vi "Is Concrete Class.vi"(0 "SG 26GHz Path Group in":refnum<class "SG 26GHz Path Group.lvclass">, 11 "error in":errorcluster) -> (4 "SG 26GHz Path Group out":refnum<class "SG 26GHz Path Group.lvclass">, 6 "Is Concrete Class?":bool, 15 "error out":errorcluster)   [LabVIEW 2023, in "RFFixtureCharact.PXI.lvlib" / "SG 26GHz Path Group.lvclass"]
uses:
  SG 26GHz Path Group.lvclass
  SG 26GHz Path Group.lvclass/SG 26GHz Path Group.ctl
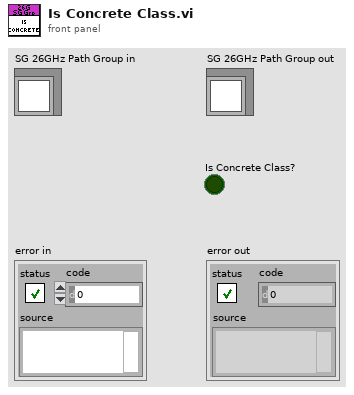
[diagram p1: front panel]
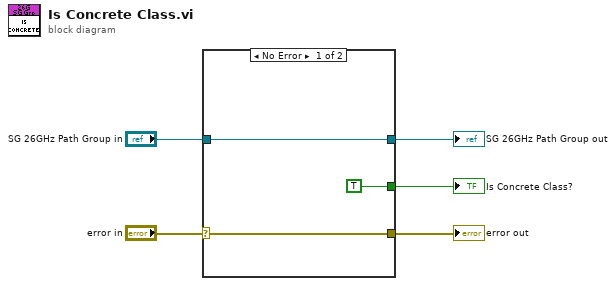
[diagram p0: block diagram]
diagram:
  n1 = case shown="No Error" "error in" {
    selector: "error in" -> [w7 w10]
    tunnel: [TRUE ("Is Concrete Class?") _] -> w1
    tunnel: [w7 w10] -> w2
    tunnel: "SG 26GHz Path Group in" -> [w6 w9]
    tunnel: [w6 w9] -> w5
    frame No Error {
    }
    frame Error {
    }
  }
  "error out" <- w2
  "SG 26GHz Path Group out" <- w5
  "Is Concrete Class?" <- w1
